vi "AVQ8347 Peakserch Data.vi"(0 "VISA Session":refnum<visa-resource-name>, 5 "Error In":errorcluster) -> (14 "Copy VISA Session":refnum<visa-resource-name>, 15 "Return All Data":string, 16 "Peakserch Data":dbl[](array[numeric]) format="%.12f", 17 "Return Data Bytes":u16, 19 "Error Out":errorcluster)   [LabVIEW 2020]
doc: "This function returns the peakserch data value"
uses:
  eeb29e85-eefd-437f-8856-766ec45e3683.vi
panel:
  out "String Work":string
  # "Peakserch Data"
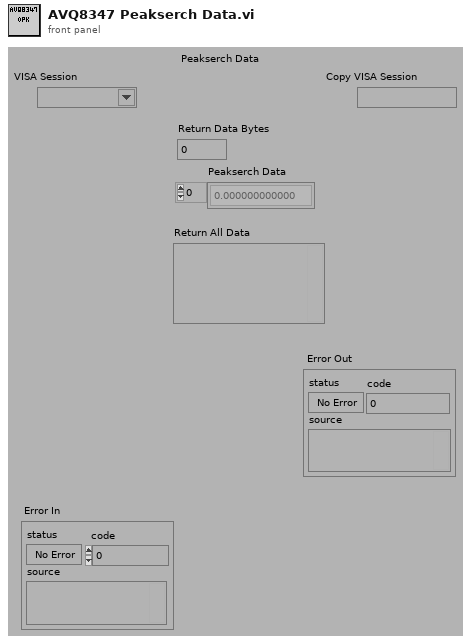
[diagram p1: front panel]
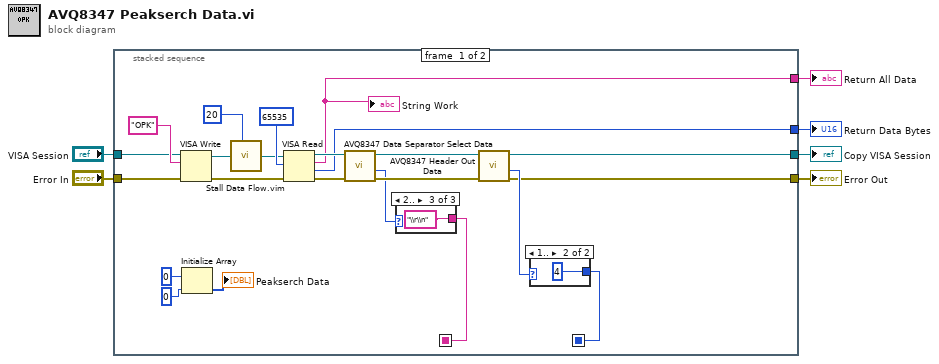
[diagram p0: block diagram]
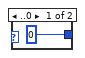
[diagram p2: hidden frame]
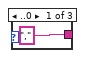
[diagram p3: hidden frame]
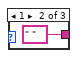
[diagram p4: hidden frame]
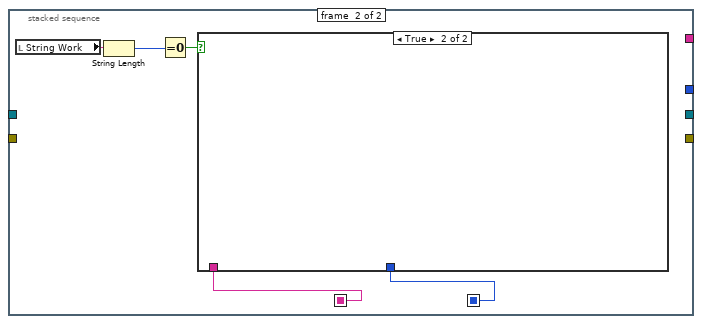
[diagram p5: hidden frame]
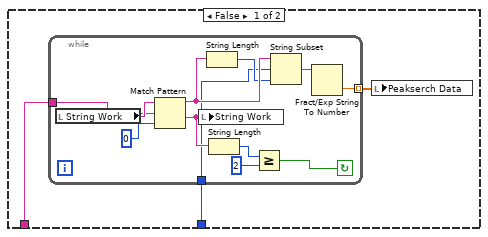
[diagram p6: hidden frame]
diagram:
  n1 = stacked-sequence {
    seq-local: [w23 _] -> [_ w36]
    seq-local: [w27 _] -> [_ w35]
    tunnel: "Error In" -> [w15 _]
    tunnel: "VISA Session" -> [w14 _]
    tunnel: [w13 _] -> w4
    tunnel: [w12 _] -> w3
    tunnel: [w11 _] -> w2
    tunnel: [w10 _] -> w1
    frame #0 {
      n2 = VISA Write(VISA resource name=w14, write buffer="OPK", error in (no error)=w15) -> (VISA resource name out=w9:refnum<visa-resource-name>, error out=w28:errorcluster)  [unwired: 1 out]
      n3 = Initialize Array(0, 0) -> (→"Peakserch Data":i32[])
      n4 = call "Stall Data Flow.vim"("value in"=w9, "milliseconds to wait"=u32 20) -> ("value out"=w8:refnum<visa-resource-name>)  [unwired: 1 out]
      n5 = VISA Read(VISA resource name=w8, byte count=65535, error in (no error)=w28) -> (VISA resource name out=w16:refnum<visa-resource-name>, read buffer=w10:string, return count=w11:u32, error out=w17:errorcluster)
      "String Work" <- w10
      n6 = call "AVQ8347 Data Separator Select Data.vi"("Error In"=w17, "VISA Session"=w16) -> ("Error Out"=w22:errorcluster, "Data Separrator Select Value"=w20:u16, "Copy VISA Session"=w21:refnum<visa-resource-name>)  [unwired: 6 in, 1 out]
      n7 = case shown="2.." w20 {
        tunnel: ["," " " "\\r\\n"] -> w23
        frame ..0 {
        }
        frame 1 {
        }
        frame 2.. {
        }
      }
      n8 = call "AVQ8347 Header Out Data.vi"("Error In"=w22, "VISA Session"=w21) -> ("Error Out"=w13:errorcluster, "Header Data Out Control Value"=w19:u16, "Copy VISA Session"=w12:refnum<visa-resource-name>)  [unwired: 6 in, 1 out]
      n9 = case shown="1.." w19 {
        tunnel: [0 4] -> w27
        frame ..0 {
        }
        frame 1.. {
        }
      }
    }
    frame #1 {
      n10 = local read "String Work"() -> (w39:string)
      n11 = String Length(string=w39) -> (length=w38:i32)
      n12 = Equal To 0?(x=w38) -> (x = 0?=w37:bool)
      n13 = case shown="True" w37 {
        tunnel: w36 -> [w41 _]
        tunnel: w35 -> [w42 _]
        frame False {
          n14 = while {
            tunnel: [w49] -> w40 mode=indexing
            tunnel: w41 -> [w48]
            tunnel: w42 -> [w43]
            stop <- w45 continue-if-true
            n15 = local read "String Work"() -> (w50:string)
            n16 = Match Pattern(string=w50, regular expression=w48, offset (0)=0) -> (before substring=w53:string, after substring=w51:string)  [unwired: 2 out]
            n17 = local write "String Work"(w51) -> ()
            n18 = String Length(string=w53) -> (length=w52:i32)
            n19 = String Length(string=w51) -> (length=w46:i32)
            n20 = Greater Or Equal?(x=w46, y=2) -> (x >= y?=w45:bool)
            n21 = String Subset(string=w53, offset (0)=w43, length (rest)=w52) -> (substring=w54:string)
            n22 = Fract/Exp String To Number(string=w54) -> (number=w49:dbl)  [unwired: 3 in, 1 out]
          }
          n23 = local write "Peakserch Data"(w40) -> ()
        }
        frame True {
        }
      }
    }
  }
  "Return Data Bytes" <- w2
  "Return All Data" <- w1
  "Error Out" <- w4
  "Copy VISA Session" <- w3
